vi "Create Pattern Script(FSN).vi"(8 "error in (no error)":errorcluster, 10 "FSN":u8, 11 "BML Pattern Creater in":refnum<class "BML Pattern Creater.lvclass">) -> (0 "error out":errorcluster, 2 "String":string, 3 "BML Pattern Creater out":refnum<class "BML Pattern Creater.lvclass">)   [LabVIEW 2018, in "BML Pattern Creater.lvlib" / "BML Pattern Creater.lvclass"]
uses:
  BML Pattern Creater.lvclass
  Interfaces/Protocol Interface.lvlibp/Interfaces/Protocol Interface/Pin State.ctl
  Interfaces/Protocol Interface.lvlibp/Interfaces/Protocol Interface/Protocol Interface.lvclass
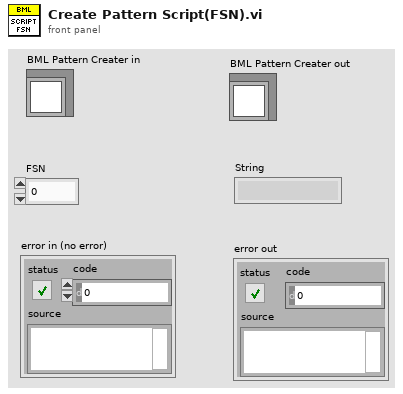
[diagram p1: front panel]
types:
  T1 = typedef "Protocol Interface.lvlibp/Protocol Interface.lvclass/Pin State.ctl" = enum16{"0", "1", "L", "H", "X", "V", "D", "M"}
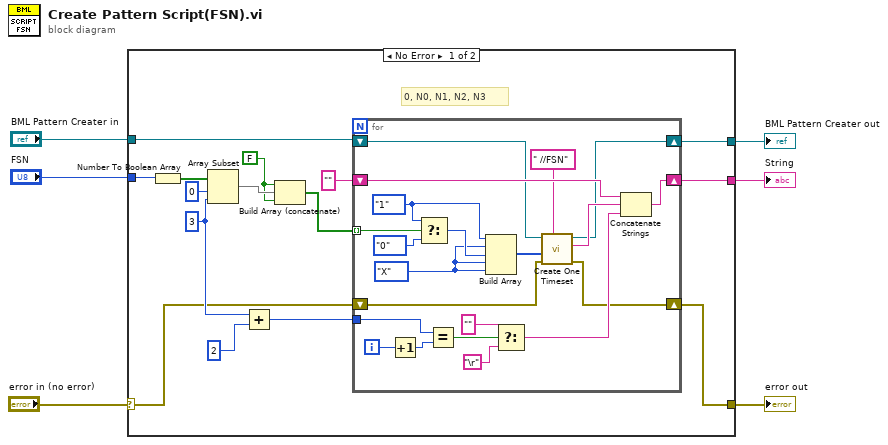
[diagram p0: block diagram]
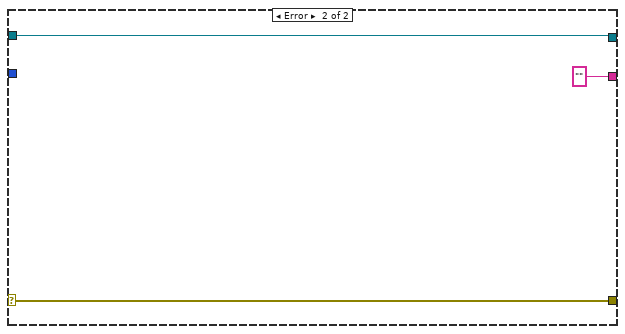
[diagram p2: hidden frame]
diagram:
  n1 = case shown="No Error" "error in (no error)" {
    selector: "error in (no error)" -> [w10 w44]
    tunnel: [w11 ""] -> w5
    tunnel: [w9 w44] -> w4
    tunnel: "FSN" -> [w21 _]
    tunnel: "BML Pattern Creater in" -> [w8 w43]
    tunnel: [w7 w43] -> w1
    frame No Error {
      w16 = FALSE
      w14 = 3 ("length")
      # "0, N0, N1, N2, N3"
      n2 = Number To Boolean Array(number=w21) -> (Boolean array=w20:bool[])
      n3 = Array Subset(array=w20, index=0, length=w14) -> (w17:bool[])
      n4 = Add(x=w14, y=2) -> (x+y=w12:i32)
      n5 = Build Array (concatenate)(w16, w17, w16) -> (w15:bool[])
      n6 = for {
        tunnel: w12 -> [w40]
        shift-right: [w35] -> w11
        shift-left: "" -> [w34]
        tunnel: w15 -> [w33] mode=indexing
        shift-right: [w24] -> w9
        shift-left: w10 -> [w25]
        shift-right: [w22] -> w7
        shift-left: w8 -> [w23]
        i -> [w42]
        w28 = Pin_State."X" ("PinState")
        w30 = Pin_State."1" ("PinState")
        n7 = Increment(x=w42) -> (x+1=w41:i32)
        n8 = Select(t=w30, s=w33, f=Pin_State."0" ("PinState")) -> (s? t:f=w32:T1)
        n9 = Equal?(x=w40, y=w41) -> (x = y?=w39:bool)
        n10 = Build Array(w30, w28, w32, w28, w28) -> (w31:T1[])
        n11 = Select(t="", s=w39, f="\r") -> (s? t:f=w36:string)
        n12 = call-dynamic "Create One Timeset.vi"("Notes"=" //FSN", "error in (no error)"=w25, "Pin State"=w31, "BML Pattern Creater in"=w23) -> ("error out"=w24:errorcluster, "string out"=w26:string, "BML Pattern Creater out"=w22:refnum<class "BML Pattern Creater.lvclass">)  [unwired: 5 in]
        n13 = Concatenate Strings(w34, w26, w36) -> (w35:string)
      }
    }
    frame Error {
    }
  }
  "String" <- w5
  "error out" <- w4
  "BML Pattern Creater out" <- w1
